vi "CommInitialize.vi"(8 "error in (no error)":errorcluster, 11 "DMA_Write In":refnum<class "DMA_Write.lvclass">) -> (0 "error out":errorcluster, 3 "Node*":refnum<data-value>)   [LabVIEW 2013, in "DMA_Write.lvclass"]
uses:
  DMA_Write.lvclass
  xCE/xceNode/xceNode.lvclass
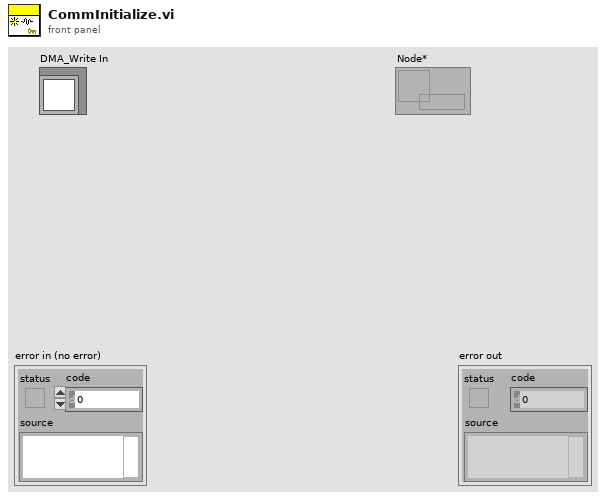
[diagram p1: front panel]
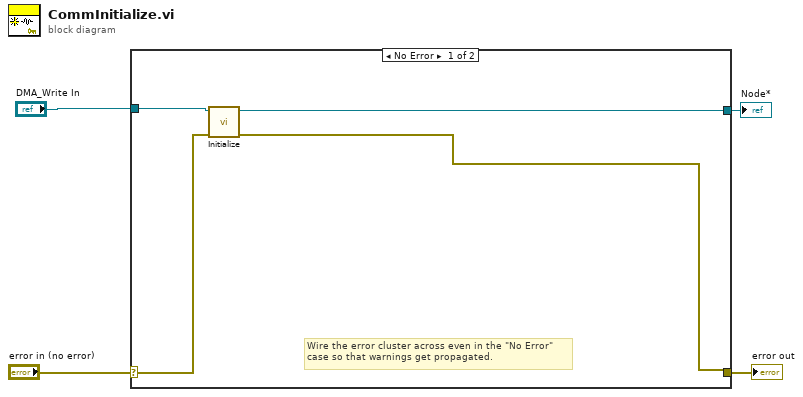
[diagram p0: block diagram]
diagram:
  n1 = case shown="No Error" "error in (no error)" {
    selector: "error in (no error)" -> [w7 w9]
    tunnel: [w5 w9] -> w4
    tunnel: "DMA_Write In" -> [w8 _]
    tunnel: [w6 _] -> w2
    frame No Error {
      # "Wire the error cluster across even in the \"No Error\"\ncase so that warnings get propagated."
      n2 = call-dynamic "Initialize.vi"("error in"=w7, "DMA_Write in"=w8) -> ("error out"=w5:errorcluster, "Node*"=w6:refnum<data-value>)  [unwired: 8 in]
    }
    frame Error {
    }
  }
  "error out" <- w4
  "Node*" <- w2
